vi "Text to Double.vi"(11 "string":string) -> (3 "number":dbl)   [LabVIEW 2018]
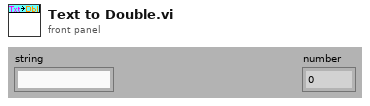
[diagram p1: front panel]
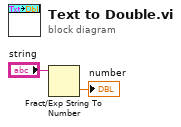
[diagram p0: block diagram]
diagram:
  n1 = Fract/Exp String To Number(string="string") -> (number=→"number":dbl)  [unwired: 3 in, 1 out]
